vi "T7_Read_FLOAT32_Register.vi"(9 "LabJack TestFLOAT32 Register":u16=55124, 10 "Remote Port":u16=502, 11 "Remote IP Address":string="192.168.1.15") -> (6 "Raw Data Read":u16[](array[numeric]), 7 "Read FLOAT32":sgl)   [LabVIEW 2014]
uses:
  Serial Link Layer/NI_Modbus_Cleaned/NI Modbus121Clean.llb/MB Ethernet Master Query Read Input Registers (poly).vi
panel:
  # "MB Ethernet Example Master.vi\n\nInstructions\n1.Use Kipling to find your devices IP address & modify the\n\"Remote IP Addres\"\n2. Run this VI\n3. Change value of \"FLOAT32 to Write\" & press \"Write Data\""
  # "TCP Parameters"
  # "Test Write & Read of TEST_UINT32 Register"
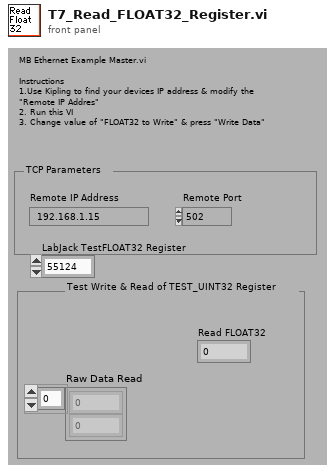
[diagram p1: front panel]
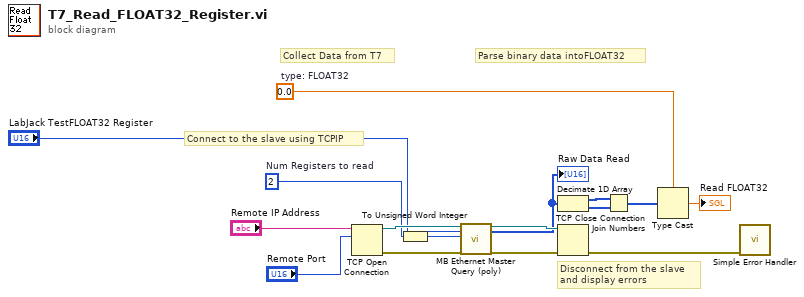
[diagram p0: block diagram]
diagram:
  w3 = sgl 0.0  # type: FLOAT32
  w8 = 2  # Num Registers to read
  # "Parse binary data intoFLOAT32"
  # "Collect Data from T7"
  # "Disconnect from the slave\nand display errors"
  # "Connect to the slave using TCPIP"
  n1 = TCP Open Connection(address="Remote IP Address", remote port or service name="Remote Port") -> (connection ID=w14:refnum<k5>, error out=w13:errorcluster)  [unwired: 3 in]
  n2 = To Unsigned Word Integer(number=w8) -> (unsigned 16bit integer=w1:u16)
  n3 = call-poly "MB Ethernet Master Query (poly).vi"("TCP Connection Refnum in"=w14, "Starting Address"="LabJack TestFLOAT32 Register", "Quantity"=w1, "error in"=w13) -> ("TCP Connection Refnum (dup)"=w10:refnum<k5>, "Input Registers"=w5:u16[], "error out"=w11:errorcluster)  [unwired: 12 in, 1 out]
  "Raw Data Read" <- w5
  n4 = Decimate 1D Array(w5) -> (w7:u16[], w6:u16[])
  n5 = TCP Close Connection(connection ID=w10, error in (no error)=w11) -> (error out=w12:errorcluster)  [unwired: 2 out]
  n6 = Join Numbers(hi=w7, lo=w6) -> ((hi.lo)=w4:u32[])
  n7 = Type Cast(type=w3, x=w4) -> (*(type *) &x=→"Read FLOAT32":sgl)
  n8 = call <vilib>:"Simple Error Handler.vi"("error in (no error)"=w12) -> ()  [unwired: 1 in, 8 out]
